vi "KE6221 -- Set Wave Type.vi"(0 "Resource In":refnum<visa-resource-name>, 1 "Check For SCPI Errors? (T)":bool=TRUE, 7 "Wave Type":T1, 11 "error in (no error)":errorcluster) -> (4 "Resource Out (dupl)":refnum<visa-resource-name>, 15 "error out":errorcluster)   [LabVIEW 2019, in "Keithley 622x.lvlib"]
uses:
  Keithley 622x.lvlib
  Low Level/Typedefs/KE6221 -- Wave Type.ctl
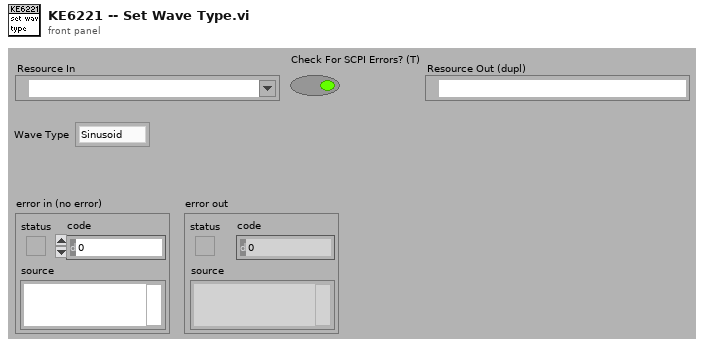
[diagram p1: front panel]
types:
  T1 = typedef "Keithley 622x.lvlib/KE6221 -- Wave Type.ctl" = enum16{"Sinusoid", "Square", "Ramp", "Arbitrary 0", "Arbitrary 1", "Arbitrary 2", "Arbitrary 3", "Arbitrary 4"}
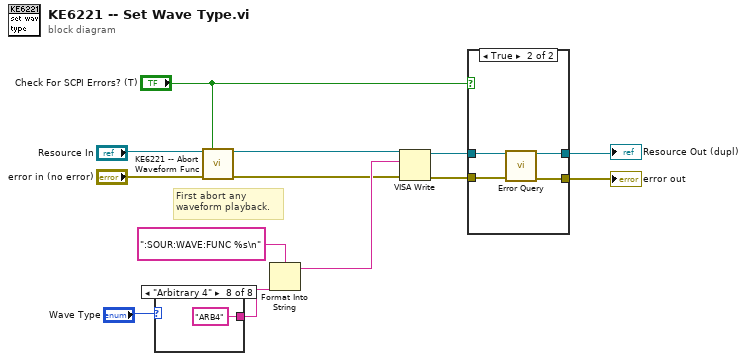
[diagram p0: block diagram]
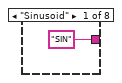
[diagram p2: hidden frame]
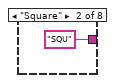
[diagram p3: hidden frame]
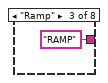
[diagram p4: hidden frame]
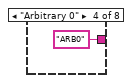
[diagram p5: hidden frame]
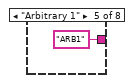
[diagram p6: hidden frame]
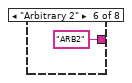
[diagram p7: hidden frame]
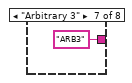
[diagram p8: hidden frame]
diagram:
  # "First abort any\nwaveform playback."
  n1 = case shown="\"Arbitrary 4\"" "Wave Type" {
    tunnel: ["SIN" "SQU" "RAMP" "ARB0" "ARB1" "ARB2" "ARB3" "ARB4"] -> w8
    frame "Sinusoid" {
    }
    frame "Square" {
    }
    frame "Ramp" {
    }
    frame "Arbitrary 0" {
    }
    frame "Arbitrary 1" {
    }
    frame "Arbitrary 2" {
    }
    frame "Arbitrary 3" {
    }
    frame "Arbitrary 4" {
    }
  }
  n2 = call "KE6221 -- Abort Waveform Func.vi"("Resource In"="Resource In", "Check For SCPI Errors? (T)"="Check For SCPI Errors? (T)", "error in (no error)"="error in (no error)") -> ("Resource Out (dupl)"=w4:refnum<visa-resource-name>, "error out"=w3:errorcluster)  [unwired: 11 in]
  n3 = Format Into String(format string=":SOUR:WAVE:FUNC %s\n", w8) -> (resulting string=w12:string)  [unwired: 2 in, 1 out]
  n4 = VISA Write(VISA resource name=w4, write buffer=w12, error in (no error)=w3) -> (VISA resource name out=w11:refnum<visa-resource-name>, error out=w10:errorcluster)  [unwired: 1 out]
  n5 = case shown="True" "Check For SCPI Errors? (T)" {
    tunnel: w11 -> [w23 w27]
    tunnel: w10 -> [w22 w26]
    tunnel: [w22 w25] -> w1
    tunnel: [w23 w24] -> w2
    frame False {
    }
    frame True {
      n6 = call "Error Query.vi"("VISA Resource In"=w27, "error in (no error)"=w26) -> ("VISA Resource Out (dupl)"=w24:refnum<visa-resource-name>, "error out"=w25:errorcluster)  [unwired: 10 in, 2 out]
    }
  }
  "Resource Out (dupl)" <- w2
  "error out" <- w1
